vi "RT-Shutter-Main.vi"(8 "error in (no error)":errorcluster) -> (0 "error out":errorcluster)   [LabVIEW 2016]
uses:
  Controls/Shutters.ctl
  Controls/Shutter Data.ctl
  Controls/Shutter States.ctl
  Controls/Operational Modes.ctl
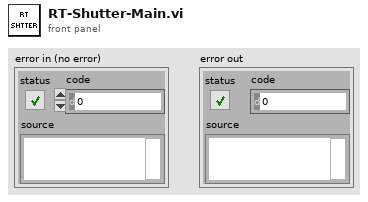
[diagram p1: front panel]
types:
  T1 = typedef "Shutters.ctl" = cluster{"Science":T2, "LFCSim":T2, "ExtendFlat":T2, "SimFlat":T2, "Solar":T2}
  T2 = typedef "Shutter Data.ctl" = cluster{"Time Stamp Control":timestamp, "State":bool, "Set":T3}
  T3 = typedef "Shutter States.ctl" = enum16{"Open", "Close", "Wait", "Off", "Arm", "Idle"}
  T4 = typedef "Operational Modes.ctl" = enum16{"Sci", "Sci-LFC", "Solar", "Solar-LFC", "LFC", "LFC-Sim", "LFC-Both", "ThAr", "ThAr-LFC", "Flat", "ExtFlat", "ExtFlat-Sim", "ExtFlat-Both", "Qtz", "ExtQtz", "ExtQtz-Sim", "ExtQtz-Both", "Dark", "Manual", "Off"}
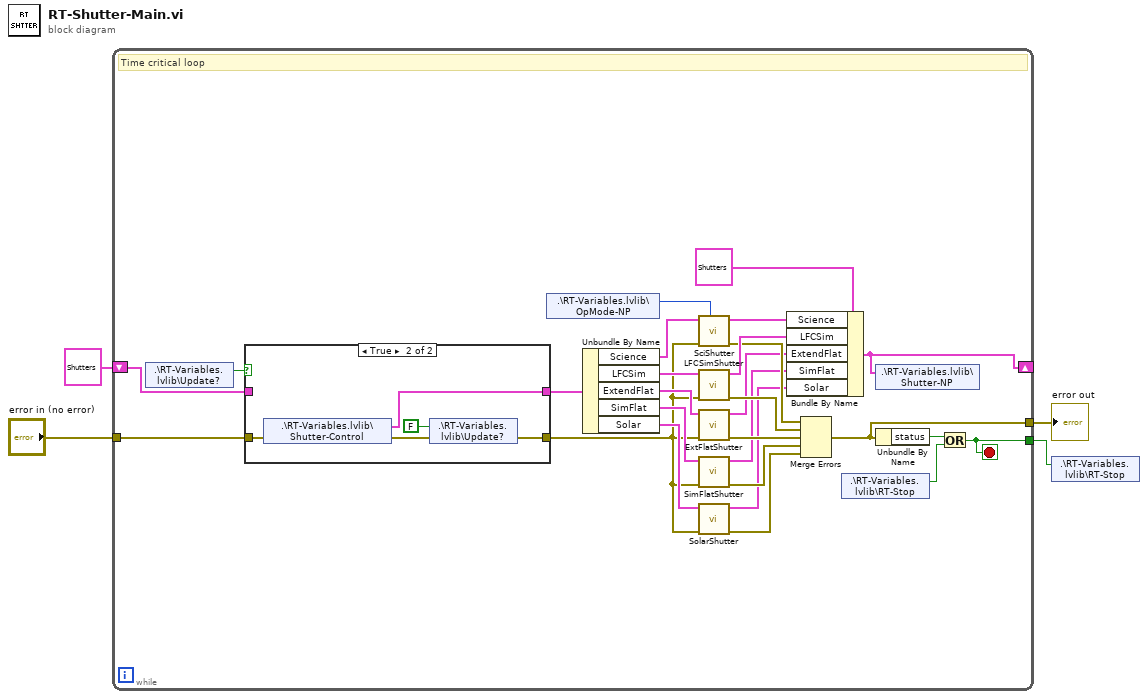
[diagram p0: block diagram]
diagram:
  n1 = while {
    tunnel: [w31] -> w1
    tunnel: "error in (no error)" -> [w27]
    tunnel: [w8] -> w2
    shift-right: [w18] -> _
    shift-left: T1 {"Science"={"Time Stamp Control"=timestamp(0 s since 1904-01-01), "State"=FALSE, "Set"=enum."Open"}, "LFCSim"={"Time Stamp Control"=timestamp(0 s since 1904-01-01), "State"=FALSE, "Set"=enum."Open"}, "ExtendFlat"={"Time Stamp Control"=timestamp(0 s since 1904-01-01), "State"=FALSE, "Set"=enum."Open"}, "SimFlat"={"Time Stamp Control"=timestamp(0 s since 1904-01-01), "State"=FALSE, "Set"=enum."Open"}, "Solar"={"Time Stamp Control"=timestamp(0 s since 1904-01-01), "State"=FALSE, "Set"=enum."Open"}} ("Shutters") -> [w25]
    stop <- w31 stop-if-true
    # "Time critical loop"
    n2 = shared-variable ".\\RT-Variables.lvlib\\Update?"() -> (w26:bool)  [unwired: 1 in, 1 out]
    n3 = case shown="True" w26 {
      tunnel: w27 -> [w32 w35]
      tunnel: w25 -> [w33 _]
      tunnel: [w33 w37] -> w23
      tunnel: [w32 w34] -> w14
      frame False {
      }
      frame True {
        n4 = shared-variable ".\\RT-Variables.lvlib\\Shutter-Control"(error in=w35) -> (w37:T1, error out=w36:errorcluster)
        n5 = shared-variable ".\\RT-Variables.lvlib\\Update?"(FALSE ("Update?"), error in=w36) -> (error out=w34:errorcluster)
      }
    }
    n6 = shared-variable ".\\RT-Variables.lvlib\\OpMode-NP"() -> (w29:T4)  [unwired: 1 in, 1 out]
    n7 = Unbundle By Name(w23) -> ("Science"=w22:T2, "LFCSim"=w19:T2, "ExtendFlat"=w17:T2, "SimFlat"=w16:T2, "Solar"=w15:T2)
    n8 = call "SciShutter.vi"("Operational Mode"=w29, "error in (no error)"=w14, "Science"=w22) -> ("error out"=w13:errorcluster, "Science out"=w24:T2)  [unwired: 6 in, 1 out]
    n9 = call "LFCSimShutter.vi"("error in (no error)"=w14, "LFCSim"=w19) -> ("error out"=w12:errorcluster, "LFCSim out"=w21:T2)  [unwired: 8 in]
    n10 = call "ExtFlatShutter.vi"("error in (no error)"=w14, "ExtFlat"=w17) -> ("error out"=w11:errorcluster, "ExtFlat out"=w7:T2)  [unwired: 8 in]
    n11 = call "SimFlatShutter.vi"("error in (no error)"=w14, "SimFlat"=w16) -> ("error out"=w10:errorcluster, "SimFlat out"=w6:T2)  [unwired: 8 in]
    n12 = call "SolarShutter.vi"("error in (no error)"=w14, "Solar"=w15) -> ("error out"=w9:errorcluster, "Solar out"=w5:T2)  [unwired: 8 in]
    n13 = Bundle By Name(cluster=T1 {"Science"={"Time Stamp Control"=timestamp(0 s since 1904-01-01), "State"=FALSE, "Set"=enum."Open"}, "LFCSim"={"Time Stamp Control"=timestamp(0 s since 1904-01-01), "State"=FALSE, "Set"=enum."Open"}, "ExtendFlat"={"Time Stamp Control"=timestamp(0 s since 1904-01-01), "State"=FALSE, "Set"=enum."Open"}, "SimFlat"={"Time Stamp Control"=timestamp(0 s since 1904-01-01), "State"=FALSE, "Set"=enum."Open"}, "Solar"={"Time Stamp Control"=timestamp(0 s since 1904-01-01), "State"=FALSE, "Set"=enum."Open"}} ("Shutters"), "Science"=w24, "LFCSim"=w21, "ExtendFlat"=w7, "SimFlat"=w6, "Solar"=w5) -> (w18:T1)
    n14 = Merge Errors(w13, w12, w11, w10, w9) -> (w8:errorcluster)
    n15 = shared-variable ".\\RT-Variables.lvlib\\RT-Stop"() -> (w30:bool)  [unwired: 1 in, 1 out]
    n16 = shared-variable ".\\RT-Variables.lvlib\\Shutter-NP"(w18) -> ()  [unwired: 1 in, 1 out]
    n17 = Unbundle By Name(w8) -> ("status"=w28:bool)
    n18 = Or(x=w28, y=w30) -> (x .or. y?=w31:bool)
  }
  "error out" <- w2
  n19 = shared-variable ".\\RT-Variables.lvlib\\RT-Stop"(w1) -> ()  [unwired: 1 in, 1 out]
